vi "Ex4 arms.vi"() -> ()   [LabVIEW 2013]
uses:
  ROS/Code/JointPositions.ctl
panel:
  in  "Joint Positions":T1 {"w2" scale=-175.25..175.25; "w1" scale=-90.0..120.0; "w0" scale=-175.25..175.25; "e1" scale=-3.0..150.0; "e0" scale=-173.5..173.5; "s1" scale=-123.0..60.0; "s0" scale=-141.0..51.0}
  in  "stop":bool
  # "Control Baxter's Arms using the supplied Position Controller"
  # "Currently fails to open /robot/limb/right/command_joint_angles due to issue 2 - Multiple Publishers in Loop \n(https://github.com/chris-smith/ROSforLabview/issues/2)"
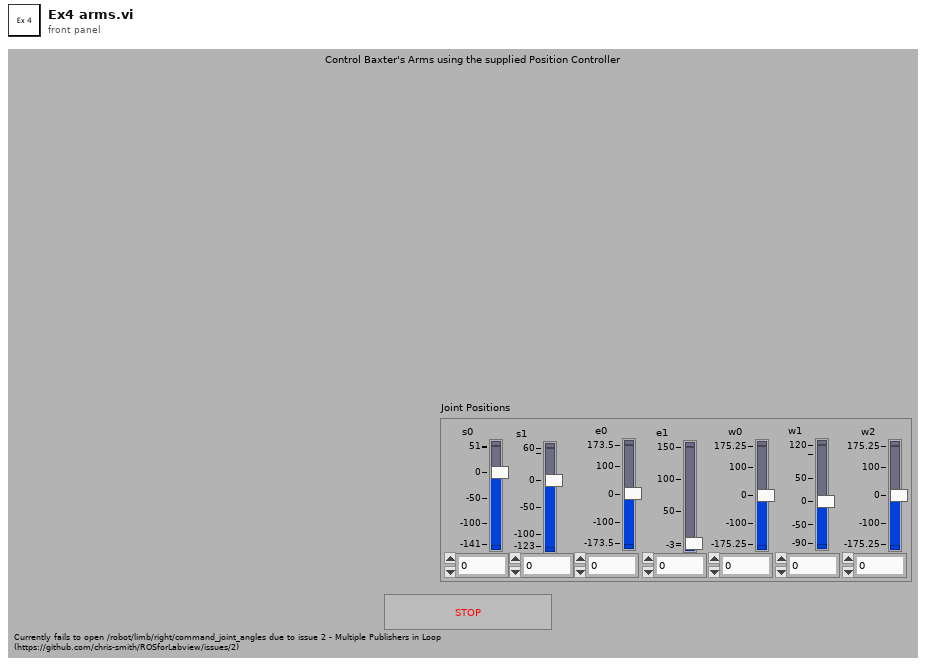
[diagram p1: front panel]
types:
  T1 = typedef "JointPositions.ctl" = cluster{"e0":dbl, "e1":dbl, "s0":dbl, "s1":dbl, "w0":dbl, "w1":dbl, "w2":dbl}
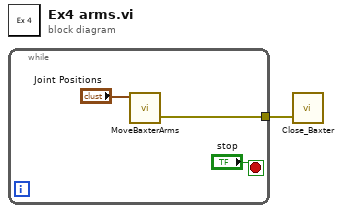
[diagram p0: block diagram]
diagram:
  n1 = while {
    tunnel: [w2] -> w1
    stop <- "stop" stop-if-true
    n2 = call "MoveBaxterArms.vi"("Left"="Joint Positions") -> ("error out"=w2:errorcluster)  [unwired: 5 in]
  }
  n3 = call "Close_Baxter.vi"("error in"=w1) -> ()  [unwired: 3 in, 1 out]
